vi "basic - VL Receive 2 VL.vi"() -> ()   [LabVIEW 2020]
uses:
  _controls/comm_computedMAC-IP.ctl
  _controls/comm_verification_rx.ctl
  _controls/comm_udp_rx.ctl
  _polimorphicInstances/session/Fdx Create Session (Rx-VL-Oriented).vi
  bsp/AFDX_Receive/Fdx Create Rx VL.vi
  _polimorphicInstances/udpPort/Fdx Create UDP Port (RX-CommPort).vi
  _polimorphicInstances/control/Fdx Start (Rx).vi
  _polimorphicInstances/control/Fdx Stop (Rx).vi
  _polimorphicInstances/session/Fdx Close Session (Port).vi
  AIM664LV.lvlib
panel:
  out "MsgCount 2":u32
  out "MsgErrorCount 2":u32
  out "MsgErrorCount":u32
  out "MsgCount":u32
  out "MsgRead 2":u32
  out "MsgRead":u32
  out "computedAddresses 2":T1 {"MACsrc" format="%.0x"}
  in  "CommPort Config 2":T2={"PortType"=enum."FDX_UDP_SAMPLING", "SubVIId"=1, "domainID"=1, "sideID"=1, "locationID"=1, "partitionID"=1, "UdpSrcPort"=12345, "UdpDstPort"=12346, "UdpNumBufMessages"=0, "UdpMaxMessageSize"=1000, "UdpSamplingRate"=128} {"partitionID" format="%.0b"}
  out "Data 2":u8[](array[numeric])
  in  "PortMap":u32
  out "Data":u8[](array[numeric])
  in  "CommPort Config 1":T2={"PortType"=enum."FDX_UDP_SAMPLING", "SubVIId"=1, "domainID"=1, "sideID"=1, "locationID"=1, "partitionID"=1, "UdpSrcPort"=12345, "UdpDstPort"=12346, "UdpNumBufMessages"=0, "UdpMaxMessageSize"=1000, "UdpSamplingRate"=128} {"partitionID" format="%.0b"}
  in  "VL Config":T3={"VlId"=60, "VLRange"=1, "VerificationMode"=0, "Bag"=0, "Jitter"=0, "MaxFrameLength"=0, "MaxSkew"=0, "VLBufSize"=32768, "FilterMode"=0, "FilterPosition"=0, "Padding"=0, "FilterMask"=0, "FilterData"=0, "MinFrameLength"=0} {"FilterMode" items=["FDX_RX_VL_FLT_DIS", "FDX_RX_VL_FLT_ENA ", "FDX_RX_VL_FLT_ENA_INV"]; "MaxFrameLength" format="%.0x"; "VerificationMode" items=["FDX_RX_VL_CHECK_ENA_DEFAULT"=65535, "FDX_RX_VL_CHECK_REDMAM"=16, "DX_RX_VL_CHECK_TRAFIC"=8, "FDX_RX_VL_CHECK_FRAMESIZE"=4, "FDX_RX_VL_CHECK_SNINTEG"=2, "FDX_RX_VL_CHECK_INVPAC"=1, "FDX_RX_VL_CHECK_DISA"=0]}
  in  "DefaultPayloadMode (Full)":u32(ring) items=["FDX_PAYLOAD_FULL", "FDX_PAYLOAD_IP_EXT", "FDX_PAYLOAD_IP", "FDX_PAYLOAD_MAC"]
  out "read time uS":cluster{u32, u32}(graph)
  in  "Port":u32=1
  in  "Board":u32
  out "current time":timestamp
  out "current irig time":T4={"SignOut"=-1509901600, "DayOut"=16, "HourOut"=8, "MinOut"=7, "SecondOut"=53, "MilliSecOut"=368, "MicroSecOut"=508, "NanoSecOut"=600, "InfoOut"=0, "Mode"=3}
  out "computedAddresses 1":T1 {"MACsrc" format="%.0x"}
  in  "stop":bool
  out "PortInitOut":T5 {"PortConfig" items=["FDX_SINGLE", "FDX_REDUNDANT"]}
  out "error out":errorcluster
  # "ARINC 664 - Receiving through VL (Virtual Link)"
  # "Overview: Setup the board to transmit package as raw frames.\nRequirement: One AIM ARINC-664 board with installed AIM ARINC 664 BSP.\nRestrictions: None.\nInstruction:\n1. Select the Board ID (0 if you have only one board in your system) and the port number. If you want to validate between two ports in one device, you can use tx board and Rx Board\n2. Run the VI.\n3. See the result in Current IRIG Time"
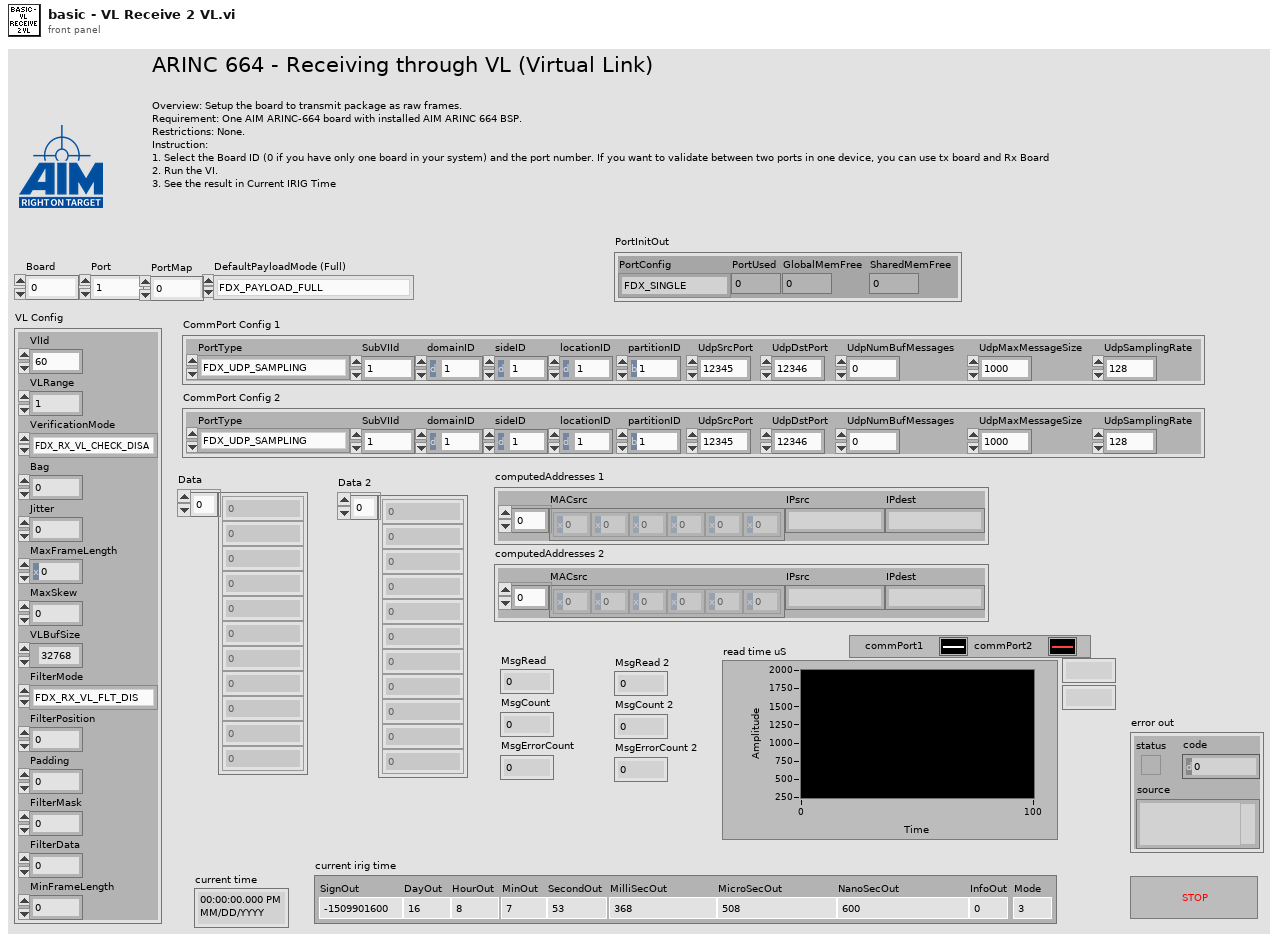
[diagram p1: front panel]
types:
  T1 = typedef "AIM664LV.lvlib/comm_computedMAC-IP.ctl" = cluster{"MACsrc":u8[], "IPsrc":string, "IPdest":string}
  T2 = typedef "AIM664LV.lvlib/comm_udp_rx.ctl" = cluster{"PortType":enum16{"FDX_UDP_SAMPLING", "FDX_UDP_QUEUING"}, "SubVIId":u32, "domainID":u8, "sideID":u8, "locationID":u8, "partitionID":u8, "UdpSrcPort":u16, "UdpDstPort":u16, "UdpNumBufMessages":u32, "UdpMaxMessageSize":u32, "UdpSamplingRate":u32}
  T3 = typedef "AIM664LV.lvlib/comm_verification_rx.ctl" = cluster{"VlId":u16, "VLRange":u32, "VerificationMode":u32, "Bag":u32, "Jitter":u32, "MaxFrameLength":u32, "MaxSkew":u32, "VLBufSize":u32, "FilterMode":u32, "FilterPosition":u32, "Padding":u32, "FilterMask":u32, "FilterData":u32, "MinFrameLength":u32}
  T4 = cluster{"SignOut":i32, "DayOut":u32, "HourOut":u32, "MinOut":u32, "SecondOut":u32, "MilliSecOut":u32, "MicroSecOut":u32, "NanoSecOut":u32, "InfoOut":u32, "Mode":u32}
  T5 = cluster{"PortConfig":u32, "PortUsed":u32, "GlobalMemFree":u32, "SharedMemFree":u32}
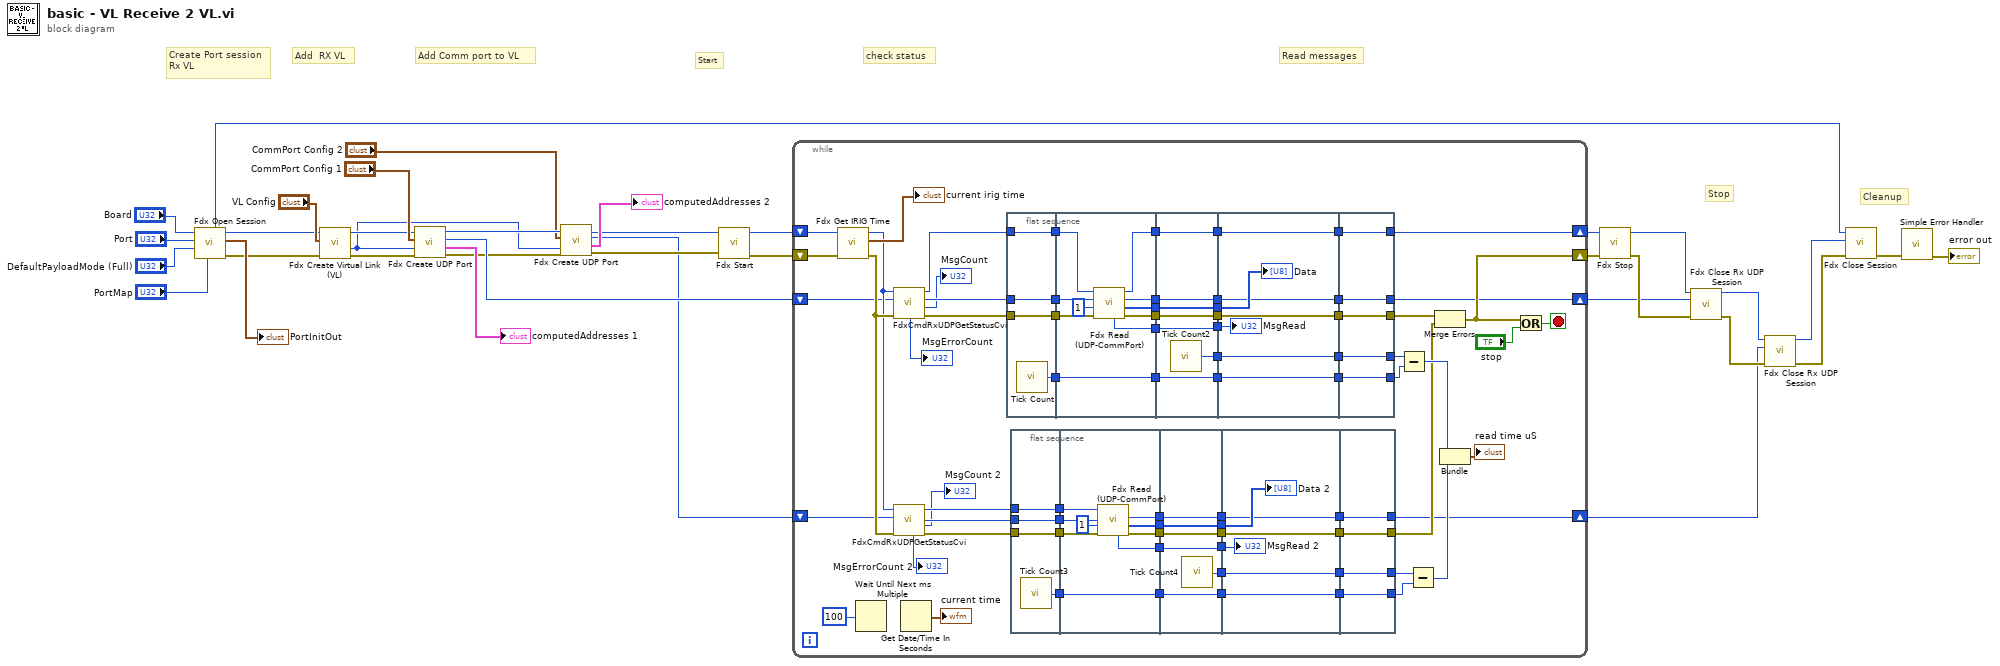
[diagram p0: block diagram]
diagram:
  # "Cleanup"
  # "Stop"
  # "Read messages"
  # "check status"
  # "Start"
  # "Add Comm port to VL"
  # "Add  RX VL"
  # "Create Port session\nRx VL"
  n1 = call-poly "Fdx Open Session.vi"("PortMap"="PortMap", "DefaultPayloadMode (Full)"="DefaultPayloadMode (Full)", "port"="Port", "board"="Board") -> ("error out"=w24:errorcluster, "PortInitOut"=→"PortInitOut":T5, "InstrumentHandle_port out"=w25:u32, "InstrumentHandle_board out"=w5:u32)  [unwired: 2 in, 2 out]
  n2 = call-poly "Fdx Create Virtual Link (VL).vi"("error in (no error)"=w24, "VL Config"="VL Config", "InstrumentHandle_port in"=w25) -> ("error out"=w27:errorcluster, "VlId"=w14:u16, "InstrumentHandle_port out"=w26:u32)  [unwired: 6 in]
  n3 = call-poly "Fdx Create UDP Port.vi"("error in"=w27, "VlId"=w14, "CommPort Config"="CommPort Config 1", "port handle in"=w26) -> ("error out"=w17:errorcluster, "computedAddresses"=→"computedAddresses 1":T1, "commPort handle out"=w21:u32, "port handle out"=w16:u32)  [unwired: 4 in]
  n4 = call-poly "Fdx Create UDP Port.vi"("error in"=w17, "VlId"=w14, "CommPort Config"="CommPort Config 2", "port handle in"=w16) -> ("error out"=w12:errorcluster, "computedAddresses"=→"computedAddresses 2":T1, "commPort handle out"=w6:u32, "port handle out"=w11:u32)  [unwired: 4 in]
  n5 = call-poly "Fdx Start.vi"("error in"=w12, "InstrumentHandle_port in"=w11) -> ("error out"=w35:errorcluster, "InstrumentHandle_port out"=w34:u32)  [unwired: 8 in]
  n6 = while {
    shift-right: [w92] -> w36
    shift-left: w34 -> [w108]
    shift-right: [w62] -> w22
    shift-left: w35 -> [w107]
    shift-right: [w40] -> w3
    shift-left: w21 -> [w49]
    shift-right: [w44] -> w4
    shift-left: w6 -> [w50]
    stop <- w110 stop-if-true
    n7 = call "Fdx Get IRIG Time.vi"("error in (no error)"=w107, "InstrumentHandle_board in"=w108) -> ("error out"=w55:errorcluster, "Curent Irig Time"=→"current irig time":T4, "InstrumentHandle_board out"=w51:u32)  [unwired: 7 in]
    n8 = Wait Until Next ms Multiple(millisecond multiple=u32 100) -> ()  [unwired: 1 out]
    n9 = call "FdxCmdRxUDPGetStatusCvi.vi"("error in"=w55, "UdpHandle"=w49, "InstrumentHandle_port"=w51) -> ("error out"=w56:errorcluster, "MsgCount"=→"MsgCount":u32, "UdpHandle Out"=w57:u32, "InstrumentHandle_port"=w58:u32, "MsgErrorCount"=→"MsgErrorCount":u32)  [unwired: 4 in]
    n10 = call "FdxCmdRxUDPGetStatusCvi.vi"("error in"=w55, "UdpHandle"=w50, "InstrumentHandle_port"=w51) -> ("error out"=w54:errorcluster, "MsgCount"=→"MsgCount 2":u32, "UdpHandle Out"=w53:u32, "InstrumentHandle_port"=w52:u32, "MsgErrorCount"=→"MsgErrorCount 2":u32)  [unwired: 4 in]
    n11 = Get Date/Time In Seconds() -> (seconds since 1Jan1904=→"current time":timestamp)
    n12 = flat-sequence {
      tunnel: w56 -> [w144]
      tunnel: [w144] -> w101
      tunnel: [w143] -> w100
      tunnel: w58 -> [w142]
      tunnel: [w142] -> w93
      tunnel: w57 -> [w141]
      tunnel: [w141] -> w87
      tunnel: w101 -> [w153]
      tunnel: [w152] -> w99
      tunnel: w100 -> [w154]
      tunnel: [w154] -> w97
      tunnel: w93 -> [w151]
      tunnel: [w150] -> w89
      tunnel: w87 -> [w149]
      tunnel: [w148] -> w85
      tunnel: [w147] -> w67
      tunnel: [w146] -> w37
      tunnel: w99 -> [w161]
      tunnel: [w161] -> w98
      tunnel: w97 -> [w160]
      tunnel: [w160] -> w96
      tunnel: [w159] -> w94
      tunnel: [w158] -> w90
      tunnel: w89 -> [w158]
      tunnel: [w157] -> w86
      tunnel: w85 -> [w157]
      tunnel: [w156] -> w68
      tunnel: w67 -> [w156]
      tunnel: [w155] -> w38
      tunnel: w37 -> [w155]
      tunnel: w98 -> [w165]
      tunnel: w96 -> [w168]
      tunnel: [w168] -> w103
      tunnel: [w167] -> w95
      tunnel: w94 -> [w167]
      tunnel: [w166] -> w91
      tunnel: w90 -> [w166]
      tunnel: [w165] -> w88
      tunnel: w86 -> [w164]
      tunnel: w68 -> [w163]
      tunnel: [w162] -> w39
      tunnel: w38 -> [w162]
      tunnel: [w173] -> w104
      tunnel: w103 -> [w173]
      tunnel: [w172] -> w69
      tunnel: w95 -> [w172]
      tunnel: [w171] -> w92
      tunnel: w91 -> [w171]
      tunnel: [w170] -> w84
      tunnel: w88 -> [w170]
      tunnel: [w169] -> w40
      tunnel: w39 -> [w169]
      frame #0 {
        n13 = call "Tick Count"() -> ("Tick Count(uSec)"=w143:u32)
      }
      frame #1 {
        n14 = call "Fdx Read (UDP-CommPort).vi"("error in"=w153, "MsgCount"=u32 1, "UdpHandle"=w149, "InstrumentHandle_port"=w151) -> ("error out"=w152:errorcluster, "ReadBuffer"=w148:u8[], "UdpHandle  Out"=w146:u32, "InstrumentHandle_port"=w150:u32, "MsgRead"=w147:u32)  [unwired: 3 in]
      }
      frame #2 {
        n15 = call "Tick Count2"() -> ("Tick Count(uSec)"=w159:u32)
      }
      frame #3 {
        "Data" <- w164
        "MsgRead" <- w163
      }
      frame #4 {
      }
    }
    n16 = flat-sequence {
      tunnel: w54 -> [w115]
      tunnel: [w115] -> w83
      tunnel: [w114] -> w82
      tunnel: w52 -> [w113]
      tunnel: [w113] -> w81
      tunnel: w53 -> [w112]
      tunnel: [w112] -> w80
      tunnel: w83 -> [w123]
      tunnel: [w122] -> w79
      tunnel: w82 -> [w124]
      tunnel: [w124] -> w78
      tunnel: w81 -> [w121]
      tunnel: w80 -> [w120]
      tunnel: [w119] -> w77
      tunnel: [w118] -> w65
      tunnel: [w117] -> w41
      tunnel: w79 -> [w130]
      tunnel: [w130] -> w76
      tunnel: w78 -> [w129]
      tunnel: [w129] -> w75
      tunnel: [w128] -> w74
      tunnel: [w127] -> w73
      tunnel: w77 -> [w127]
      tunnel: [w126] -> w66
      tunnel: w65 -> [w126]
      tunnel: [w125] -> w42
      tunnel: w41 -> [w125]
      tunnel: w76 -> [w134]
      tunnel: w75 -> [w136]
      tunnel: [w136] -> w72
      tunnel: [w135] -> w71
      tunnel: w74 -> [w135]
      tunnel: [w134] -> w70
      tunnel: w73 -> [w133]
      tunnel: w66 -> [w132]
      tunnel: [w131] -> w43
      tunnel: w42 -> [w131]
      tunnel: [w140] -> w64
      tunnel: w72 -> [w140]
      tunnel: [w139] -> w63
      tunnel: w71 -> [w139]
      tunnel: [w138] -> w61
      tunnel: w70 -> [w138]
      tunnel: [w137] -> w44
      tunnel: w43 -> [w137]
      frame #0 {
        n17 = call "Tick Count3"() -> ("Tick Count(uSec)"=w114:u32)
      }
      frame #1 {
        n18 = call "Fdx Read (UDP-CommPort).vi"("error in"=w123, "MsgCount"=u32 1, "UdpHandle"=w120, "InstrumentHandle_port"=w121) -> ("error out"=w122:errorcluster, "ReadBuffer"=w119:u8[], "UdpHandle  Out"=w117:u32, "MsgRead"=w118:u32)  [unwired: 3 in, 1 out]
      }
      frame #2 {
        n19 = call "Tick Count4"() -> ("Tick Count(uSec)"=w128:u32)
      }
      frame #3 {
        "Data 2" <- w133
        "MsgRead 2" <- w132
      }
      frame #4 {
      }
    }
    n20 = Subtract(x=w69, y=w104) -> (x-y=w102:u32)
    n21 = Subtract(x=w63, y=w64) -> (x-y=w59:u32)
    n22 = Merge Errors(w84, w61) -> (w62:errorcluster)
    n23 = Bundle(w102, w59) -> (→"read time uS":cluster{u32, u32})  [unwired: 1 in]
    n24 = Or(x=w62, y="stop") -> (x .or. y?=w110:bool)
  }
  n25 = call-poly "Fdx Stop.vi"("error in"=w22, "InstrumentHandle_port in"=w36) -> ("error out"=w33:errorcluster, "InstrumentHandle_port out"=w20:u32)  [unwired: 8 in]
  n26 = call "Fdx Close Rx UDP Session.vi"("error in"=w33, "UdpHandle"=w3, "InstrumentHandle_port"=w20) -> ("error out"=w10:errorcluster, "InstrumentHandle_port"=w8:u32)  [unwired: 7 in]
  n27 = call "Fdx Close Rx UDP Session.vi"("error in"=w10, "UdpHandle"=w4, "InstrumentHandle_port"=w8) -> ("error out"=w9:errorcluster, "InstrumentHandle_port"=w7:u32)  [unwired: 7 in]
  n28 = call-poly "Fdx Close Session.vi"("error in"=w9, "InstrumentHandle_port in"=w7, "InstrumentHandle_board in"=w5) -> ("error out"=w2:errorcluster)  [unwired: 8 in]
  n29 = call <vilib>:"Simple Error Handler.vi"("error in (no error)"=w2) -> ("error out"=→"error out":errorcluster)  [unwired: 4 in, 4 out]
